vi "题目2.vi"() -> ()   [LabVIEW 2017]
panel:
  out "注册":bool
  in  "簇":cluster{"学号":dbl, "名字":string, "注册":bool}
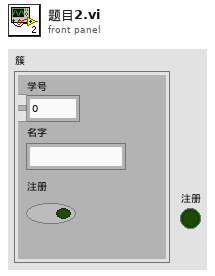
[diagram p1: front panel]
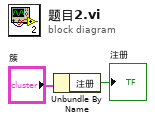
[diagram p0: block diagram]
diagram:
  n1 = Unbundle By Name("簇") -> ("注册"=→"注册":bool)
